vi "SparkTest.vi"() -> ()   [LabVIEW 2016]
uses:
  <vilib>/DAQmx/create/channels.llb/DAQmx Create Channel (CO-Pulse Generation-Frequency).vi
  <vilib>/DAQmx/configure/timing.llb/DAQmx Timing (Implicit).vi
  <resource>/objmgr/daqmx.rc
panel:
  in  "Spark":bool=TRUE
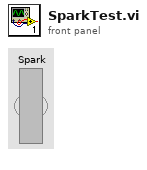
[diagram p1: front panel]
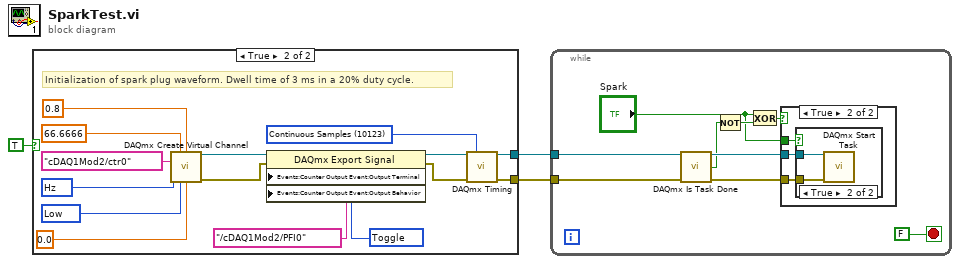
[diagram p0: block diagram]
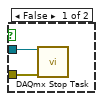
[diagram p3: hidden frame]
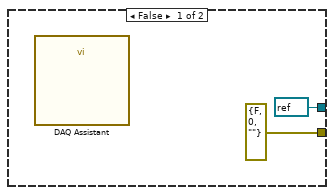
[diagram p4: hidden frame]
diagram:
  n1 = case shown="True" TRUE {
    tunnel: [errorcluster {"status"=FALSE, "code"=0, "source"=""} ("error out") w7] -> w1
    tunnel: [refnum<k21> refnum ("task out") w6] -> w2
    frame False {
      n2 = call "DAQ Assistant"() -> ()  [unwired: 18 in, 2 out]
    }
    frame True {
      w10 = 10373 items=["Hz"=10373] ("units")
      w12 = 10307 items=["Pulse"=10265, "Toggle"=10307] ("CtrOutEvent.OutputBehavior")
      w18 = 10123 items=["Finite Samples"=10178, "Continuous Samples"=10123, "Hardware Timed Single Point"=12522] ("sample mode")
      w20 = 10214 items=["High"=10192, "Low"=10214] ("idle state")
      # "Initialization of spark plug waveform. Dwell time of 3 ms in a 20% duty cycle."
      n3 = call-poly <vilib>:"DAQmx Create Virtual Channel.vi"("frequency"=66.6666, "duty cycle"=0.8, "counter"=tag "cDAQ1Mod2/ctr0", "units"=w10, "idle state"=w20, "initial delay"=0.0) -> ("task out"=w16:refnum<k21>, "error out"=w15:errorcluster)  [unwired: 8 in]
      n4 = property class="DAQmx Export Signal"(reference=w16, error in=w15, "Events:Counter Output Event:Output Terminal"=tag "/cDAQ1Mod2/PFI0" ("CtrOutEvent.OutputTerm"), "Events:Counter Output Event:Output Behavior"=w12) -> (reference out=w14:refnum<k21>, error out=w13:errorcluster)
      n5 = call-poly <vilib>:"DAQmx Timing.vi"("task/channels in"=w14, "sample mode"=w18, "error in"=w13) -> ("task out"=w6:refnum<k21>, "error out"=w7:errorcluster)  [unwired: 11 in]
    }
  }
  n6 = while {
    tunnel: w2 -> [w23]
    tunnel: w1 -> [w22]
    stop <- FALSE stop-if-true
    n7 = call <vilib>:"DAQmx Is Task Done.vi"("task/channels in"=w23, "error in"=w22) -> ("task out"=w28:refnum<k21>, "task done?"=w24:bool, "error out"=w27:errorcluster)  [unwired: 11 in]
    n8 = Not(x=w24) -> (.not. x?=w25:bool)
    n9 = Exclusive Or(1:w25, 2:"Spark") -> (0:w26:bool)
    n10 = case shown="True" w26 {
      tunnel: w28 -> [_ w32]
      tunnel: w27 -> [_ w31]
      tunnel: "Spark" -> [_ w30]
      frame False {
      }
      frame True {
        n11 = case shown="True" w30 {
          tunnel: w32 -> [w34 w36]
          tunnel: w31 -> [w33 w35]
          frame False {
            n12 = call <vilib>:"DAQmx Stop Task.vi"("task/channels in"=w34, "error in"=w33) -> ()  [unwired: 12 in, 2 out]
          }
          frame True {
            n13 = call <vilib>:"DAQmx Start Task.vi"("task/channels in"=w36, "error in"=w35) -> ()  [unwired: 12 in, 2 out]
          }
        }
      }
    }
  }
